vi "GetComparisonResult4Graphis.vi"(1 "Comparison In":T1, 8 "AND vs OR":bool) -> (15 "True?":bool)   [LabVIEW 2020]
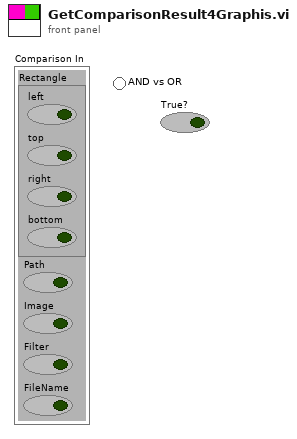
[diagram p1: front panel]
types:
  T1 = cluster{"Rectangle":cluster{"left":bool, "top":bool, "right":bool, "bottom":bool}, "Path":bool, "Image":bool, "Filter":bool, "FileName":bool}
  T2 = cluster{"left":bool, "top":bool, "right":bool, "bottom":bool}
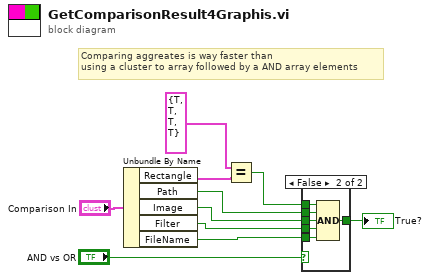
[diagram p0: block diagram]
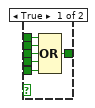
[diagram p2: hidden frame]
diagram:
  # "Comparing aggreates is way faster than\nusing a cluster to array followed by a AND array elements"
  n1 = Unbundle By Name("Comparison In") -> ("Rectangle"=w3:T2, "Path"=w6:bool, "Image"=w7:bool, "Filter"=w8:bool, "FileName"=w9:bool)
  n2 = Equal?(x=T2 {"left"=TRUE, "top"=TRUE, "right"=TRUE, "bottom"=TRUE} ("Rectangle"), y=w3) -> (x = y?=w1:bool)
  n3 = case shown="False" "AND vs OR" {
    tunnel: w9 -> [w16 w22]
    tunnel: w8 -> [w15 w21]
    tunnel: w7 -> [w14 w20]
    tunnel: w6 -> [w13 w19]
    tunnel: w1 -> [w12 w18]
    tunnel: [w11 w17] -> w5
    frame True {
      n4 = Compound Arithmetic op=OR(w12, w13, w14, w15, w16) -> (w11:bool)
    }
    frame False {
      n5 = Compound Arithmetic op=AND(w18, w19, w20, w21, w22) -> (w17:bool)
    }
  }
  "True?" <- w5
